vi "Send Read RandomNum.vi"(7 "Message Priority (Normal)":T1=enum."Normal", 8 "error in (no error)":errorcluster, 11 "Message Enqueuer":refnum<class "Message Enqueuer.lvclass">) -> (0 "error out":errorcluster, 2 "RandomNum":dbl, 3 "Message Enqueuer out":refnum<class "Message Enqueuer.lvclass">)   [LabVIEW 2014, in "Generator.lvlib" / "Read RandomNum Msg.lvclass"]
doc: "This VI sends the message to an actor."
uses:
  Read RandomNum Msg.lvclass
  <vilib>/ActorFramework/Reply Msg/Reply Msg.lvclass
  <vilib>/ActorFramework/Message Enqueuer/Message Enqueuer.lvclass
  <vilib>/ActorFramework/Message Enqueuer/Message Priority.ctl
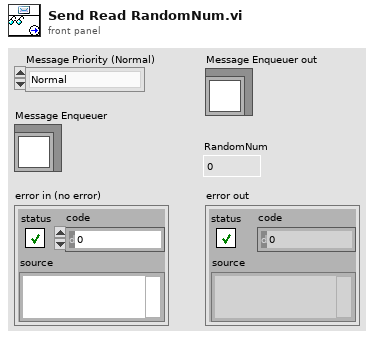
[diagram p1: front panel]
types:
  T1 = typedef "Actor Framework.lvlib/Message Enqueuer.lvclass/Message Priority.ctl" = enum16{"Low", "Normal", "High"}
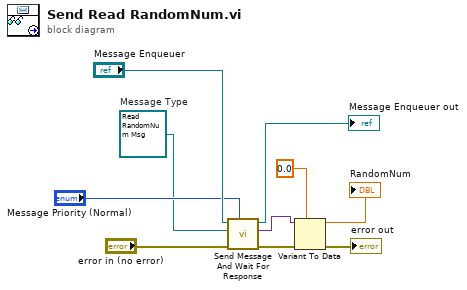
[diagram p0: block diagram]
diagram:
  w5 = refnum<class "Read RandomNum Msg.lvclass"> refnum  # Message Type
  n1 = call <vilib>:"Send Message And Wait For Response.vi"("Message Priority (Normal)"="Message Priority (Normal)", "error in (no error)"="error in (no error)", "Original Message"=w5, "Message Enqueuer in"="Message Enqueuer") -> ("error out"=w8:errorcluster, "Reply"=w3:variant, "Message Enqueuer out"=→"Message Enqueuer out":refnum<class "Message Enqueuer.lvclass">)  [unwired: 4 in, 1 out]
  n2 = Variant To Data(error in=w8, type=0.0, Variant=w3) -> (data=→"RandomNum":dbl, error out=→"error out":errorcluster)
